vi "Exec Query & Fetch.vi"(6 "scripts":string, 8 "error in":errorcluster, 11 "orm in":refnum<class "LV-ORM.lvclass">) -> (0 "error out":errorcluster, 3 "orm out":refnum<class "LV-ORM.lvclass">, 4 "recordset data":variant[][](array[variant]))   [LabVIEW 2018, in "LV-ORM.lvclass"]
uses:
  LV-ORM.lvclass
  LV-ORM.lvclass/LV-ORM.ctl
  <vilib>/addons/database/Connection.llb/Conn Execute.vi
  <vilib>/addons/database/Recordset.llb/Rec Fetch Recordset Data (R).vi
  <vilib>/addons/database/Recordset.llb/Rec Destroy - Connection.vi
  <vilib>/addons/database/NI_Database_API.lvlib
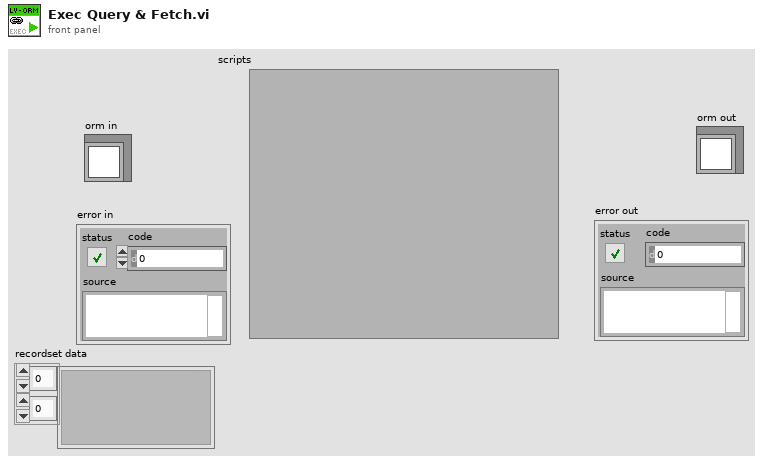
[diagram p1: front panel]
types:
  T1 = typedef "NI_Database_API.lvlib/Conn ObjectReference.ctl" = refnum<k1>
  T2 = typedef "NI_Database_API.lvlib/Rec ObjectReference.ctl" = refnum<k1>
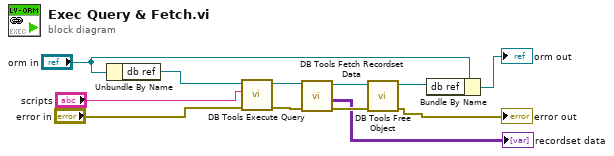
[diagram p0: block diagram]
diagram:
  n1 = Unbundle By Name("orm in") -> ("db ref"=w3:T1)
  n2 = call-poly <vilib>:"DB Tools Execute Query.vi"("error in (no error)"="error in", "SQL query"="scripts", "connection reference"=w3) -> ("error out"=w9:errorcluster, "recordset reference"=w10:T2)  [unwired: 5 in]
  n3 = call-poly <vilib>:"DB Tools Fetch Recordset Data.vi"("error in (no error)"=w9, "recordset reference"=w10) -> ("error out"=w7:errorcluster, "recordset data"=→"recordset data":variant[][], "recordset reference out"=w8:T2)  [unwired: 3 in]
  n4 = call-poly <vilib>:"DB Tools Free Object.vi"("error in (no error)"=w7, "recordset reference"=w8) -> ("error out"=→"error out":errorcluster, "connection reference"=w6:T1)  [unwired: 8 in]
  n5 = Bundle By Name(cluster="orm in", "db ref"=w6) -> (→"orm out":refnum<class "LV-ORM.lvclass">)
